vi "SW_Dispension_Calibration.vi"(8 "error in (no error)":errorcluster, 11 "Settings cluster in":T1={"Defaults"={"Default User"=0.0, "VISA Resource Name "="ASRL5::INSTR"}, "Recording and saving"={"Researcher name"="Researcher", "Name prefix"="Track", "Data post-processing"={"Filter type"=enum."Savitzky-Golay", "Length"=31, "Order"=3}, "Stop at"=0.0, "\"Stop at\" enabled"=FALSE, "Default save folder path"=path "D:/Users_Data/Dmitriy_T/Documents/MHC_Tracker", "Acquisition FPS"=enum."Max"}, "Geometry"={"Cage diameter, mm"=180, "Starting angle MIDFIELD"=0, "Starting angle BORDER"=0, "Radius, mm CENTER"=30, "Radius, mm MIDFIELD"=75, "N segments MIDFIELD"=2, "N segments BORDER"=4, "R-gap, mm"=0.0, "Bridge swap"=FALSE, "Bridge H. offset"=0.0, "Bridge V. offset"=0.0, "Twisted neck"=FALSE, "Alt. magn. orientation"=FALSE, "Sensor board size"=enum."Small"}, "IO parameters"={"IO general config."=12, "IO 1 configuration"=1, "IO 2 configuration"=1, "IO 3 configuration"=0, "IO 4 configuration"=0, "Activate ext. RS-232"=0, "IO inversion config."=0, "Sync capability"=1}, "Conditions presets array"=[{"Enabled"=FALSE, "Name"="", "Specifier(s)"=[], "Response"={"Response type"=enum."None", "TTL pulse length, ms"=0.0}}, {"Enabled"=FALSE, "Name"="", "Specifier(s)"=[], "Response"={"Response type"=enum."None", "TTL pulse length, ms"=0.0}}, {"Enabled"=FALSE, "Name"="", "Specifier(s)"=[], "Response"={"Response type"=enum."None", "TTL pulse length, ms"=0.0}}, {"Enabled"=FALSE, "Name"="", "Specifier(s)"=[], "Response"={"Response type"=enum."None", "TTL pulse length, ms"=0.0}}, {"Enabled"=FALSE, "Name"="", "Specifier(s)"=[], "Response"={"Response type"=enum."None", "TTL pulse length, ms"=0.0}}, {"Enabled"=FALSE, "Name"="", "Specifier(s)"=[], "Response"={"Response type"=enum."None", "TTL pulse length, ms"=0.0}}, {"Enabled"=FALSE, "Name"="", "Specifier(s)"=[], "Response"={"Response type"=enum."None", "TTL pulse length, ms"=0.0}}, {"Enabled"=FALSE, "Name"="", "Specifier(s)"=[], "Response"={"Response type"=enum."None", "TTL pulse length, ms"=0.0}}, {"Enabled"=FALSE, "Name"="", "Specifier(s)"=[], "Response"={"Response type"=enum."None", "TTL pulse length, ms"=0.0}}, {"Enabled"=FALSE, "Name"="", "Specifier(s)"=[], "Response"={"Response type"=enum."None", "TTL pulse length, ms"=0.0}}, {"Enabled"=FALSE, "Name"="", "Specifier(s)"=[], "Response"={"Response type"=enum."None", "TTL pulse length, ms"=0.0}}, {"Enabled"=FALSE, "Name"="", "Specifier(s)"=[], "Response"={"Response type"=enum."None", "TTL pulse length, ms"=0.0}}, {"Enabled"=FALSE, "Name"="", "Specifier(s)"=[], "Response"={"Response type"=enum."None", "TTL pulse length, ms"=0.0}}, {"Enabled"=FALSE, "Name"="", "Specifier(s)"=[], "Response"={"Response type"=enum."None", "TTL pulse length, ms"=0.0}}], "Calibration parameters"={"Timing calibration sw/hw"=0.99998266776355, "True FPS"=76.92307692307693, "True frame time, s"=80.0, "Disp. calibration info"=[]}, "Settings loaded OK"=TRUE} {"Calibration parameters"."True frame time, s" format="%.10g"; "Calibration parameters"."Disp. calibration info"."Speed, µl per ms" format="%.3g"; "Calibration parameters"."True FPS" format="%.10g"; "Calibration parameters"."Timing calibration sw/hw" format="%.10g"; "Conditions presets array"."Response"."TTL pulse length, ms" min=0.0 max=10000.0 step=10.0 format="%0.0g"; "Conditions presets array"."Specifier(s)"."Validity criteria(s)"."Validity value" min=0.0 step=0.1 format="%.2g"; "Conditions presets array"."Specifier(s)"."Value" step=1.0 format="%#.2g"; "Recording and saving"."Data post-processing"."Order" min=3 max=11 step=2; "Recording and saving"."Data post-processing"."Length" min=5 max=301 step=2; "Geometry"."Cage diameter, mm" scale=0.0..340.0}) -> (0 "error out":errorcluster, 3 "Settings cluster out":T1={"Defaults"={"Default User"=0.0, "VISA Resource Name "="ASRL5::INSTR"}, "Recording and saving"={"Researcher name"="Researcher", "Name prefix"="Track", "Data post-processing"={"Filter type"=enum."Savitzky-Golay", "Length"=31, "Order"=3}, "Stop at"=0.0, "\"Stop at\" enabled"=FALSE, "Default save folder path"=path "D:/Users_Data/Dmitriy_T/Documents/MHC_Tracker", "Acquisition FPS"=enum."Max"}, "Geometry"={"Cage diameter, mm"=180, "Starting angle MIDFIELD"=0, "Starting angle BORDER"=0, "Radius, mm CENTER"=30, "Radius, mm MIDFIELD"=75, "N segments MIDFIELD"=2, "N segments BORDER"=4, "R-gap, mm"=0.0, "Bridge swap"=FALSE, "Bridge H. offset"=0.0, "Bridge V. offset"=0.0, "Twisted neck"=FALSE, "Alt. magn. orientation"=FALSE, "Sensor board size"=enum."Small"}, "IO parameters"={"IO general config."=12, "IO 1 configuration"=1, "IO 2 configuration"=1, "IO 3 configuration"=0, "IO 4 configuration"=0, "Activate ext. RS-232"=0, "IO inversion config."=0, "Sync capability"=1}, "Conditions presets array"=[{"Enabled"=FALSE, "Name"="", "Specifier(s)"=[], "Response"={"Response type"=enum."None", "TTL pulse length, ms"=0.0}}, {"Enabled"=FALSE, "Name"="", "Specifier(s)"=[], "Response"={"Response type"=enum."None", "TTL pulse length, ms"=0.0}}, {"Enabled"=FALSE, "Name"="", "Specifier(s)"=[], "Response"={"Response type"=enum."None", "TTL pulse length, ms"=0.0}}, {"Enabled"=FALSE, "Name"="", "Specifier(s)"=[], "Response"={"Response type"=enum."None", "TTL pulse length, ms"=0.0}}, {"Enabled"=FALSE, "Name"="", "Specifier(s)"=[], "Response"={"Response type"=enum."None", "TTL pulse length, ms"=0.0}}, {"Enabled"=FALSE, "Name"="", "Specifier(s)"=[], "Response"={"Response type"=enum."None", "TTL pulse length, ms"=0.0}}, {"Enabled"=FALSE, "Name"="", "Specifier(s)"=[], "Response"={"Response type"=enum."None", "TTL pulse length, ms"=0.0}}, {"Enabled"=FALSE, "Name"="", "Specifier(s)"=[], "Response"={"Response type"=enum."None", "TTL pulse length, ms"=0.0}}, {"Enabled"=FALSE, "Name"="", "Specifier(s)"=[], "Response"={"Response type"=enum."None", "TTL pulse length, ms"=0.0}}, {"Enabled"=FALSE, "Name"="", "Specifier(s)"=[], "Response"={"Response type"=enum."None", "TTL pulse length, ms"=0.0}}, {"Enabled"=FALSE, "Name"="", "Specifier(s)"=[], "Response"={"Response type"=enum."None", "TTL pulse length, ms"=0.0}}, {"Enabled"=FALSE, "Name"="", "Specifier(s)"=[], "Response"={"Response type"=enum."None", "TTL pulse length, ms"=0.0}}, {"Enabled"=FALSE, "Name"="", "Specifier(s)"=[], "Response"={"Response type"=enum."None", "TTL pulse length, ms"=0.0}}, {"Enabled"=FALSE, "Name"="", "Specifier(s)"=[], "Response"={"Response type"=enum."None", "TTL pulse length, ms"=0.0}}], "Calibration parameters"={"Timing calibration sw/hw"=0.99998266776355, "True FPS"=76.92307692307693, "True frame time, s"=80.0, "Disp. calibration info"=[]}, "Settings loaded OK"=TRUE} {"Calibration parameters"."True frame time, s" format="%.10g"; "Calibration parameters"."Disp. calibration info"."Speed, µl per ms" format="%.3g"; "Calibration parameters"."True FPS" format="%.10g"; "Calibration parameters"."Timing calibration sw/hw" format="%.10g"; "Conditions presets array"."Response"."TTL pulse length, ms" min=0.0 max=10000.0 step=10.0 format="%0.0g"; "Conditions presets array"."Specifier(s)"."Validity criteria(s)"."Validity value" min=0.0 step=0.1 format="%.2g"; "Conditions presets array"."Specifier(s)"."Value" step=1.0 format="%#.2g"; "Recording and saving"."Data post-processing"."Order" min=3 max=11 step=2; "Recording and saving"."Data post-processing"."Length" min=5 max=301 step=2; "Geometry"."Cage diameter, mm" scale=0.0..340.0})   [LabVIEW 2018, in "Tracker.lvlib"]
uses:
  Tracker.lvlib
  Controls/CTL_Settings_cluster.ctl
  Controls/CTL_Filter_selector.ctl
  Controls/CTL_Acquisition_speed_selector.ctl
  Controls/CTL_Segmented_plot_parameters.ctl
  Controls/CTL_IO_params_cluster.ctl
  Controls/CTL_Conditions_Array.ctl
  Controls/CTL_Conditions_Cluster.ctl
  Controls/CTL_Condition_type.ctl
  Controls/CTL_Comparison_type.ctl
  Controls/CTL_Validity_check_criteria.ctl
  Controls/CTL_Condition_response_type.ctl
  Controls/CTL_Calibration_parameters.ctl
  Controls/CTL_Dispenser_calibration_info.ctl
  <vilib>/Utility/miscctls.llb/LVPointTypeDef.ctl
panel:
  out "Time spent to process command, ms":dbl
  out "Disp. calibration info":T13 {"Speed, µl per ms" format="%.3g"}
  in  "Apply":bool
  in  "Dispense":bool
  in  "Meas. vol., µl":u32=1000 max=10000 step=10
  in  "Disp. time, ms":u32=1000 max=10000 step=10
  in  "Select channel to calibrate":u16(ring) items=["Out 1"=1, "Out 2"=2]
  in  "Reset":bool
  in  "Exit":bool
  in  "Save Settings":bool
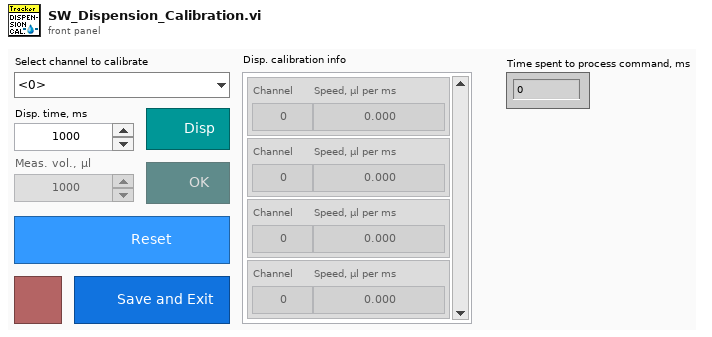
[diagram p1: front panel]
types:
  T1 = typedef "Tracker.lvlib/CTL_Settings_cluster.ctl" = cluster{"Defaults":cluster{"Default User":dbl, "VISA Resource Name ":string}, "Recording and saving":cluster{"Researcher name":string, "Name prefix":string, "Data post-processing":T2, "Stop at":dbl, "\"Stop at\" enabled":bool, "Default save folder path":path, "Acquisition FPS":T3}, "Geometry":T4, "IO parameters":T5, "Conditions presets array":T6, "Calibration parameters":T12, "Settings loaded OK":bool}
  T2 = typedef "Tracker.lvlib/CTL_Filter_selector.ctl" = cluster{"Filter type":enum16{"None", "Savitzky-Golay"}, "Length":i32, "Order":i32}
  T3 = typedef "Tracker.lvlib/CTL_Acquisition_speed_selector.ctl" = enum16{"Max", "Optimal", "Eco"}
  T4 = typedef "Tracker.lvlib/CTL_Segmented_plot_parameters.ctl" = cluster{"Cage diameter, mm":u16, "Starting angle MIDFIELD":i16, "Starting angle BORDER":i16, "Radius, mm CENTER":u16, "Radius, mm MIDFIELD":u16, "N segments MIDFIELD":u8, "N segments BORDER":u8, "R-gap, mm":sgl, "Bridge swap":bool, "Bridge H. offset":sgl, "Bridge V. offset":sgl, "Twisted neck":bool, "Alt. magn. orientation":bool, "Sensor board size":enum16{"Small", "Large"}}
  T5 = typedef "Tracker.lvlib/CTL_IO_params_cluster.ctl" = cluster{"IO general config.":u16, "IO 1 configuration":u16, "IO 2 configuration":u16, "IO 3 configuration":u16, "IO 4 configuration":u16, "Activate ext. RS-232":u16, "IO inversion config.":u16, "Sync capability":u8}
  T6 = typedef "Tracker.lvlib/CTL_Conditions_Array.ctl" = T7[]
  T7 = typedef "Tracker.lvlib/CTL_Conditions_Cluster.ctl" = cluster{"Enabled":bool, "Name":string, "Specifier(s)":cluster{"Specifier enabled":bool, "Condition type":T8, "Limit type":T9, "Value":dbl, "Validity criteria(s)":cluster{"V. check enabled":bool, "Criteria":T10, "Validity value":dbl}[]}[], "Response":cluster{"Response type":T11, "TTL pulse length, ms":dbl}}
  T8 = typedef "Tracker.lvlib/CTL_Condition_type.ctl" = enum16{"Not in use", "Speed", "Zone", "Angle to wall"}
  T9 = typedef "Tracker.lvlib/CTL_Comparison_type.ctl" = enum16{"Less", "Less or Equal", "Equal", "Greater or Equal", "Greater", "Not Equal"}
  T10 = typedef "Tracker.lvlib/CTL_Validity_check_criteria.ctl" = enum16{"Running bout (seconds)", "Running bout (meters)"}
  T11 = typedef "Tracker.lvlib/CTL_Condition_response_type.ctl" = enum16{"None", "TTL"}
  T12 = typedef "Tracker.lvlib/CTL_Calibration_parameters.ctl" = cluster{"Timing calibration sw/hw":dbl, "True FPS":dbl, "True frame time, s":dbl, "Disp. calibration info":T13}
  T13 = typedef "Tracker.lvlib/CTL_Dispenser_calibration_info.ctl" = cluster{"Channel":u8, "Speed, µl per ms":dbl}[]
  T14 = typedef "LVPointTypeDef.ctl" = cluster{"Horizontal":i16, "Vertical":i16}
  T15 = enum8{"Enabled", "Disabled", "Disabled and Grayed Out"}
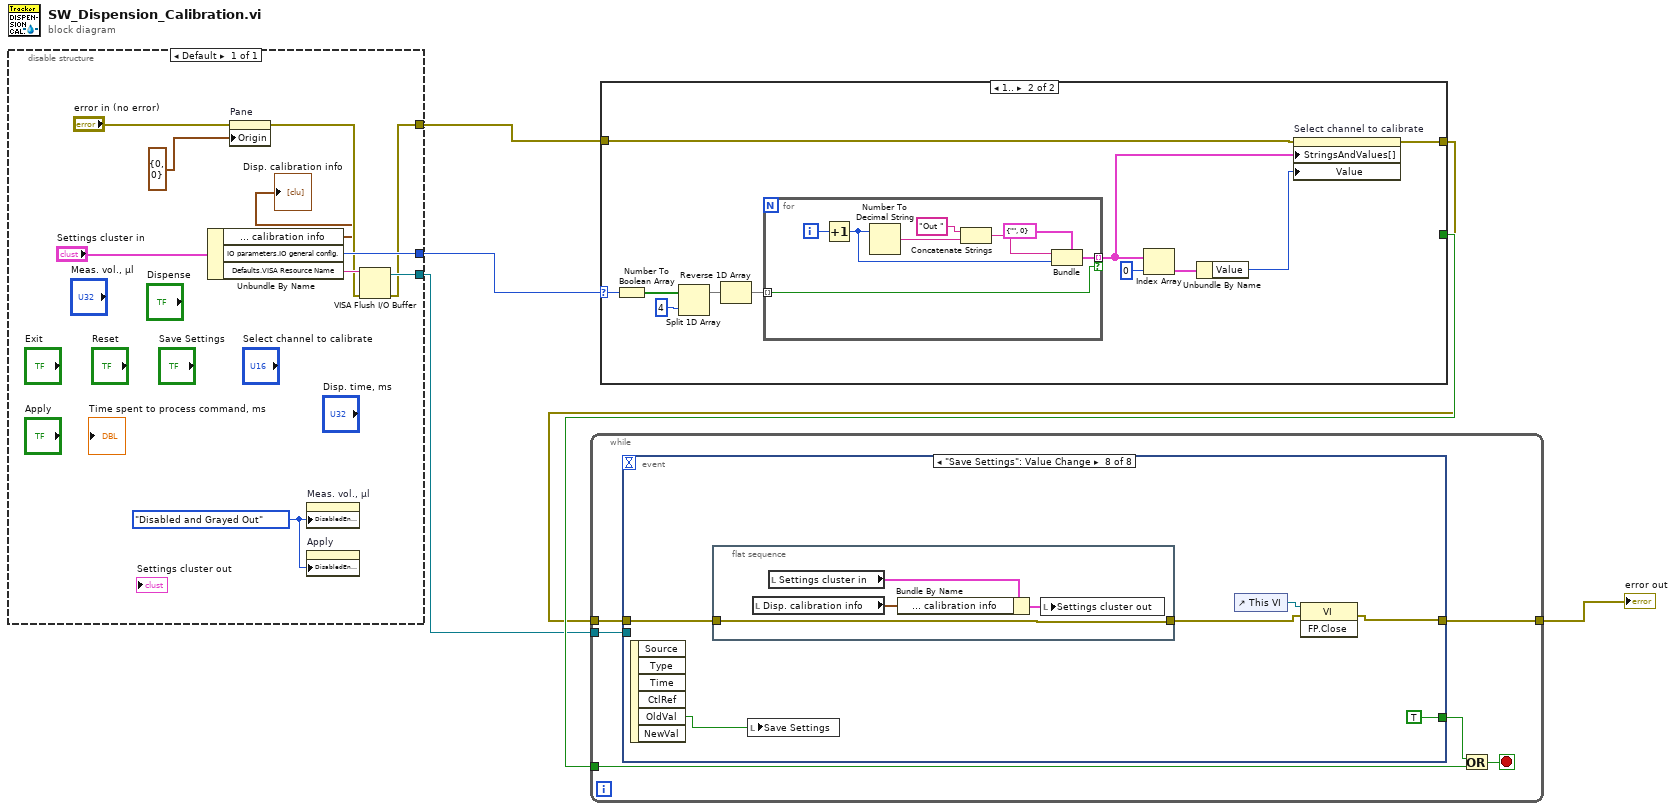
[diagram p0: block diagram]
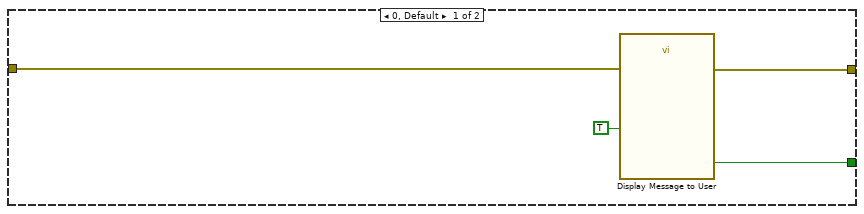
[diagram p2: hidden frame]
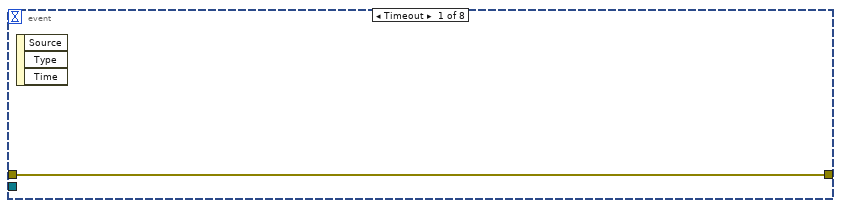
[diagram p3: hidden frame]
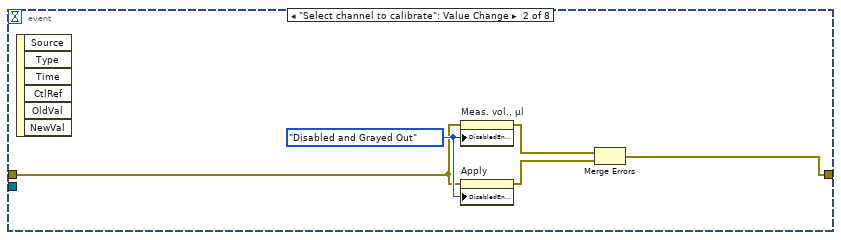
[diagram p4: hidden frame]
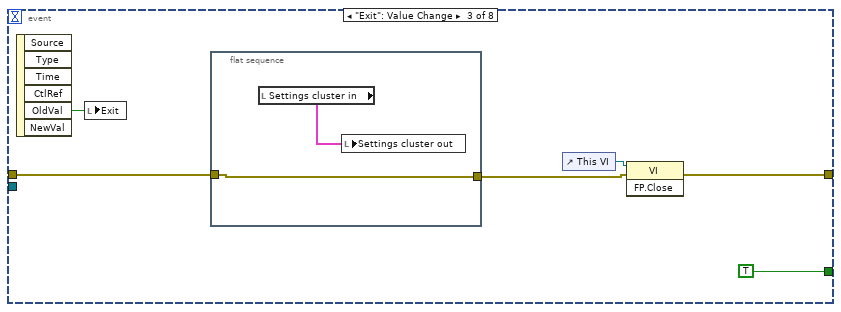
[diagram p5: hidden frame]
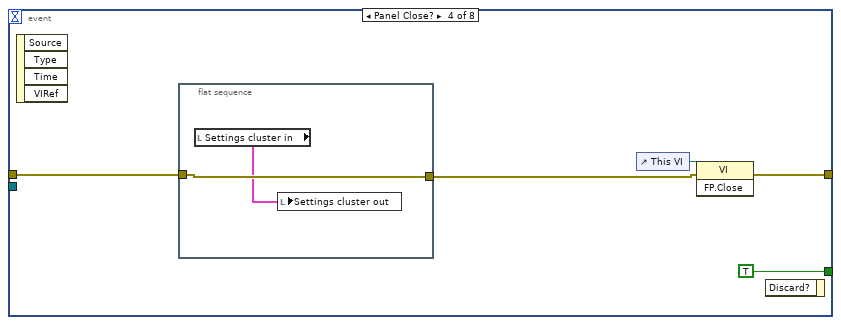
[diagram p6: hidden frame]
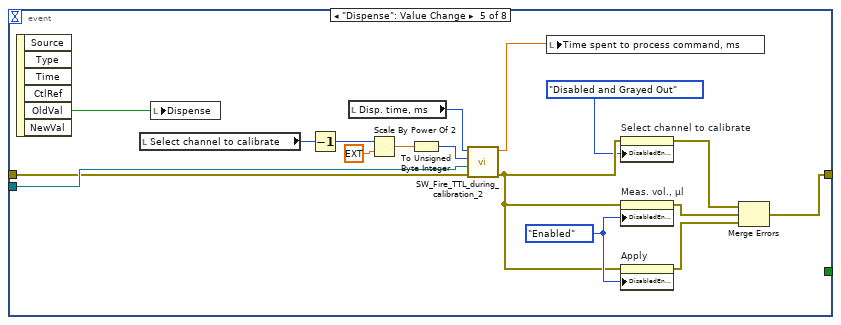
[diagram p7: hidden frame]
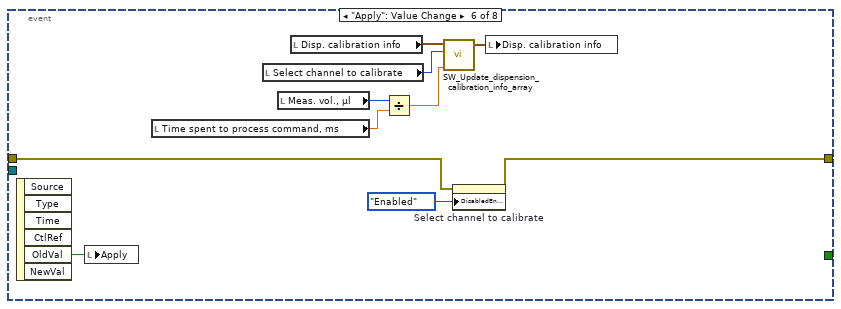
[diagram p8: hidden frame]
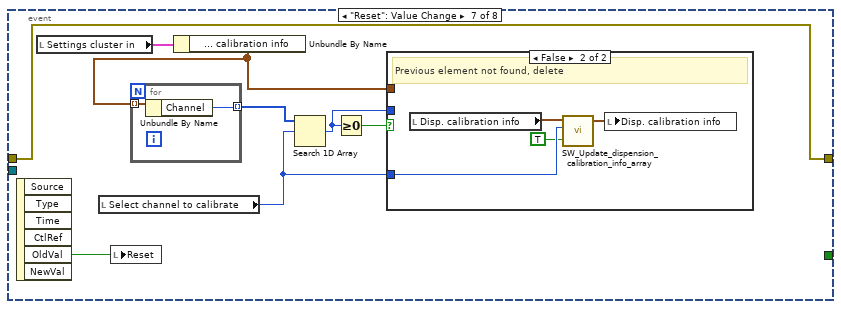
[diagram p9: hidden frame]
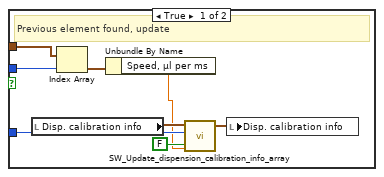
[diagram p10: hidden frame]
diagram:
  n1 = disable-structure shown="Default" {
    disable-tunnel: [w9] -> w6
    disable-tunnel: [w13] -> w5
    disable-tunnel: [w11] -> w2
    frame Enabled {
      w7 = T15."Disabled and Grayed Out" ("Disabled")
      n2 = Unbundle By Name("Settings cluster in") -> ("Calibration parameters.Disp. calibration info"=→"Disp. calibration info":T13, "IO parameters.IO general config."=w13:u16, "Defaults.VISA Resource Name"=w12:string)
      n3 = property on="Pane" class="Pane"(error in="error in (no error)", "Origin"=T14 {"Horizontal"=0, "Vertical"=0}) -> (error out=w10:errorcluster)  [unwired: 1 in, 1 out]
      n4 = property on="Meas. vol., µl" class="DigNum (strict)"("DisabledEnum"=w7) -> ()  [unwired: 2 in, 2 out]
      n5 = property on="Apply" class="Bool (strict)"("DisabledEnum"=w7) -> ()  [unwired: 2 in, 2 out]
      n6 = VISA Flush I/O Buffer(VISA resource name=w12, error in (no error)=w10) -> (VISA resource name out=w11:refnum<visa-resource-name>, error out=w9:errorcluster)  [unwired: 1 in]
    }
  }
  n7 = case shown="1.." w5 {
    selector: w5 -> [_ w27]
    tunnel: w6 -> [w19 w26]
    tunnel: [w18 w25] -> w3
    tunnel: [w17 _] -> w4
    frame 0, Default {
      n8 = call "Display Message to User"("error in (no error)"=w19, "Enable"=TRUE) -> ("error out"=w18:errorcluster, "Exit"=w17:bool)  [unwired: 8 in]
    }
    frame 1.. {
      n9 = Number To Boolean Array(number=w27) -> (Boolean array=w31:bool[])
      n10 = Split 1D Array(array=w31, index=4) -> (first subarray=w29:bool[])  [unwired: 1 out]
      n11 = Reverse 1D Array(array=w29) -> (reversed array=w28:bool[])
      n12 = for {
        tunnel: w28 -> [w34] mode=indexing
        tunnel: [w35] -> w24 mode=indexing if=w34
        i -> [w33]
        n13 = Increment(x=w33) -> (x+1=w32:i32)
        n14 = Number To Decimal String(number=w32) -> (decimal integer string=w39:string)  [unwired: 1 in]
        n15 = Concatenate Strings("Out " ("string"), w39) -> (w37:string)
        n16 = Bundle(cluster=cluster{"String":string, "Value":u8} {"String"="", "Value"=0}, "String"=w37, "Value"=w32) -> (w35:cluster{"String":string, "Value":u8})
      }
      n17 = Index Array(array=w24, index=0) -> (element=w22:cluster{"String":string, "Value":u8})
      n18 = Unbundle By Name(w22) -> ("Value"=w21:u8)
      n19 = property on="Select channel to calibrate" class="Ring (strict)"(error in=w26, "StringsAndValues[]"=w24, "Value"=w21) -> (error out=w25:errorcluster)  [unwired: 1 in, 1 out]
    }
  }
  n20 = while {
    tunnel: w4 -> [w44]
    tunnel: w3 -> [w43]
    tunnel: [w42] -> w1
    tunnel: w2 -> [w40]
    stop <- w45 stop-if-true
    n21 = event shown="[7] \"Save Settings\": Value Change" {
      selector: _ -> [_ _ _ _ _ _ _ _]
      dyn-events: _ -> [_ _ _ _ _ _ _ _]
      timeout: _ -> [_ _ _ _ _ _ _ _]
      tunnel: w43 -> [w46 w50 w53 w61 w81 w86 w99 w121]
      tunnel: [w46 w47 w54 w63 w70 w85 w99 w118] -> w42
      tunnel: [_ _ TRUE ("OldVal") TRUE ("OldVal") _ _ _ TRUE ("OldVal")] -> w41
      tunnel: w40 -> [_ _ _ _ w82 _ _ _]
      event Timeout {
        n22 = event-data() -> ()  [unwired: 1 in, 3 out]
      }
      event "Select channel to calibrate": Value Change {
        w51 = T15."Disabled and Grayed Out" ("Disabled")
        n23 = event-data() -> ()  [unwired: 1 in, 6 out]
        n24 = property on="Meas. vol., µl" class="DigNum (strict)"(error in=w50, "DisabledEnum"=w51) -> (error out=w49:errorcluster)  [unwired: 1 in, 1 out]
        n25 = property on="Apply" class="Bool (strict)"(error in=w50, "DisabledEnum"=w51) -> (error out=w48:errorcluster)  [unwired: 1 in, 1 out]
        n26 = Merge Errors(w49, w48) -> (w47:errorcluster)
      }
      event "Exit": Value Change {
        n27 = event-data() -> ("OldVal"=w56:bool)  [unwired: 1 in, 5 out]
        n28 = local write "Exit"(w56) -> ()
        n29 = flat-sequence {
          tunnel: w53 -> [w58]
          tunnel: [w58] -> w52
          frame #0 {
            n30 = local read "Settings cluster in"() -> (w59:T1)
            n31 = local write "Settings cluster out"(w59) -> ()
          }
        }
        n32 = control-ref of="This VI"() -> (w57:refnum<vi>)
        n33 = invoke class="VI" method="FP.Close"(reference=w57, error in=w52) -> (error out=w54:errorcluster)  [unwired: 1 in, 2 out]
      }
      event Panel Close? {
        n34 = event-data() -> ()  [unwired: 1 in, 4 out]
        n35 = flat-sequence {
          tunnel: w61 -> [w66]
          tunnel: [w66] -> w60
          frame #0 {
            n36 = local read "Settings cluster in"() -> (w65:T1)
            n37 = local write "Settings cluster out"(w65) -> ()
          }
        }
        n38 = control-ref of="This VI"() -> (w64:refnum<vi>)
        n39 = invoke class="VI" method="FP.Close"(reference=w64, error in=w60) -> (error out=w63:errorcluster)  [unwired: 1 in, 2 out]
        n40 = event-data() -> ()  [unwired: 2 in, 1 out]
      }
      event "Dispense": Value Change {
        w73 = T15."Enabled" ("Disabled")
        n41 = event-data() -> ("OldVal"=w83:bool)  [unwired: 1 in, 5 out]
        n42 = local read "Select channel to calibrate"() -> (w76:u16)
        n43 = local write "Dispense"(w83) -> ()
        n44 = Decrement(x=w76) -> (x-1=w75:u16)
        n45 = local read "Disp. time, ms"() -> (w79:u32)
        n46 = Scale By Power Of 2(n=w75, x=ext 1.0) -> (x*2^n=w78:ext)
        n47 = To Unsigned Byte Integer(number=w78) -> (unsigned 8bit integer=w74:u8)
        n48 = call "SW_Fire_TTL_during_calibration_2.vi"("error in (no error)"=w81, "VISA resource in"=w82, "Port to fire"=w74, "TTL pulse length, ms"=w79) -> ("error out"=w69:errorcluster, "Time spent to process command, ms"=w80:dbl)  [unwired: 5 in, 1 out]
        n49 = local write "Time spent to process command, ms"(w80) -> ()
        n50 = property on="Select channel to calibrate" class="Ring (strict)"(error in=w69, "DisabledEnum"=T15."Disabled and Grayed Out" ("Disabled")) -> (error out=w67:errorcluster)  [unwired: 1 in, 1 out]
        n51 = property on="Meas. vol., µl" class="DigNum (strict)"(error in=w69, "DisabledEnum"=w73) -> (error out=w72:errorcluster)  [unwired: 1 in, 1 out]
        n52 = property on="Apply" class="Bool (strict)"(error in=w69, "DisabledEnum"=w73) -> (error out=w71:errorcluster)  [unwired: 1 in, 1 out]
        n53 = Merge Errors(w67, w72, w71) -> (w70:errorcluster)
      }
      event "Apply": Value Change {
        n54 = event-data() -> ("OldVal"=w93:bool)  [unwired: 1 in, 5 out]
        n55 = local write "Apply"(w93) -> ()
        n56 = local read "Time spent to process command, ms"() -> (w91:dbl)
        n57 = local read "Select channel to calibrate"() -> (w88:u16)
        n58 = local read "Meas. vol., µl"() -> (w92:u32)
        n59 = local read "Disp. calibration info"() -> (w89:T13)
        n60 = Divide(x=w92, y=w91) -> (x/y=w87:dbl)
        n61 = call "SW_Update_dispension_calibration_info_array.vi"("Speed, ul per ms (10)"=w87, "Channel to update"=w88, "Disp. calibration info IN"=w89) -> ("Disp. calibration info OUT"=w90:cluster{"Channel":u8, "Speed, µl per ms":dbl}[])  [unwired: 3 in]
        n62 = property on="Select channel to calibrate" class="Ring (strict)"(error in=w86, "DisabledEnum"=T15."Enabled" ("Disabled")) -> (error out=w85:errorcluster)  [unwired: 1 in, 1 out]
        n63 = local write "Disp. calibration info"(w90) -> ()
      }
      event "Reset": Value Change {
        n64 = event-data() -> ("OldVal"=w101:bool)  [unwired: 1 in, 5 out]
        n65 = local read "Settings cluster in"() -> (w100:T1)
        n66 = local read "Select channel to calibrate"() -> (w96:u16)
        n67 = local write "Reset"(w101) -> ()
        n68 = Unbundle By Name(w100) -> ("Calibration parameters.Disp. calibration info"=w95:T13)
        n69 = for {
          tunnel: w95 -> [w115] mode=indexing
          tunnel: [w114] -> w98 mode=indexing
          n70 = Unbundle By Name(w115) -> ("Channel"=w114:u8)
        }
        n71 = Search 1D Array(1D array=w98, element=w96) -> (index of element=w94:i32)  [unwired: 1 in]
        n72 = Greater Or Equal To 0?(x=w94) -> (x >= 0?=w97:bool)
        n73 = case shown="False" w97 {
          tunnel: w96 -> [w107 w111]
          tunnel: w95 -> [w105 _]
          tunnel: w94 -> [w104 _]
          frame True {
            # "Previous element found, update"
            n74 = local read "Disp. calibration info"() -> (w109:T13)
            n75 = Index Array(array=w105, index=w104) -> (element=w103:cluster{"Channel":u8, "Speed, µl per ms":dbl})
            n76 = Unbundle By Name(w103) -> ("Speed, µl per ms"=w102:dbl)
            n77 = call "SW_Update_dispension_calibration_info_array.vi"("Speed, ul per ms (10)"=w102, "Delete channel? (F)"=FALSE, "Channel to update"=w107, "Disp. calibration info IN"=w109) -> ("Disp. calibration info OUT"=w108:cluster{"Channel":u8, "Speed, µl per ms":dbl}[])  [unwired: 2 in]
            n78 = local write "Disp. calibration info"(w108) -> ()
          }
          frame False {
            # "Previous element not found, delete"
            n79 = local read "Disp. calibration info"() -> (w113:T13)
            n80 = call "SW_Update_dispension_calibration_info_array.vi"("Delete channel? (F)"=TRUE, "Channel to update"=w111, "Disp. calibration info IN"=w113) -> ("Disp. calibration info OUT"=w112:cluster{"Channel":u8, "Speed, µl per ms":dbl}[])  [unwired: 3 in]
            n81 = local write "Disp. calibration info"(w112) -> ()
          }
        }
      }
      event "Save Settings": Value Change {
        n82 = event-data() -> ("OldVal"=w117:bool)  [unwired: 1 in, 5 out]
        n83 = flat-sequence {
          tunnel: w121 -> [w122]
          tunnel: [w122] -> w119
          frame #0 {
            n84 = local read "Disp. calibration info"() -> (w124:T13)
            n85 = local read "Settings cluster in"() -> (w125:T1)
            n86 = Bundle By Name(cluster=w125, "Calibration parameters.Disp. calibration info"=w124) -> (w123:T1)
            n87 = local write "Settings cluster out"(w123) -> ()
          }
        }
        n88 = local write "Save Settings"(w117) -> ()
        n89 = control-ref of="This VI"() -> (w120:refnum<vi>)
        n90 = invoke class="VI" method="FP.Close"(reference=w120, error in=w119) -> (error out=w118:errorcluster)  [unwired: 1 in, 2 out]
      }
    }
    n91 = Or(x=w41, y=w44) -> (x .or. y?=w45:bool)
  }
  "error out" <- w1
